vi "Verify Person as JSON.vi"(8 "error in":errorcluster) -> (0 "error out":errorcluster)   [LabVIEW 2020]
uses:
  Common/Person/Person.lvclass
  Common/Person/Person.lvclass/Person.ctl
  <vilib>/addons/_JKI Toolkits/Caraya/classes/Test/Test.lvclass
  <vilib>/SAS/Approval Tests/Extensions/Caraya.Extension/lib_Caraya.Extension.lvlib
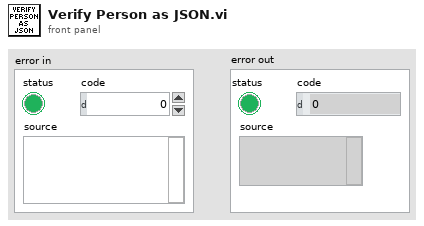
[diagram p1: front panel]
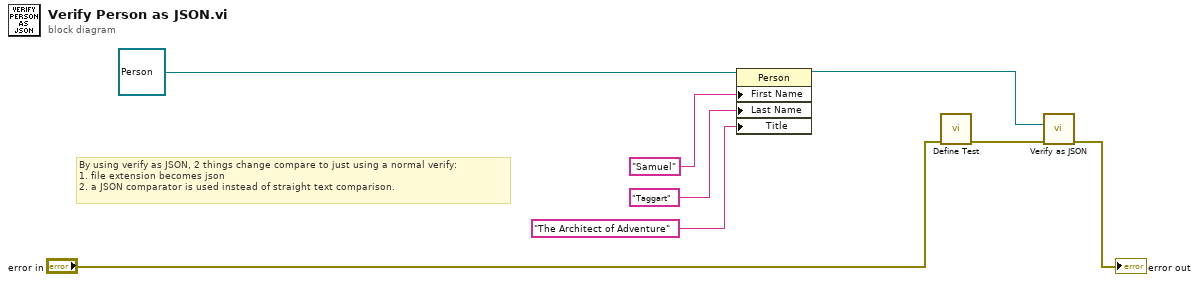
[diagram p0: block diagram]
diagram:
  # "By using verify as JSON, 2 things change compare to just using a normal verify:\n1. file extension becomes json\n2. a JSON comparator is used instead of straight text comparison."
  n1 = property class="Person"(reference=refnum<class "Person.lvclass"> refnum ("Person.lvclass"), "First Name"="Samuel", "Last Name"="Taggart", "Title"="The Architect of Adventure") -> (reference out=w1:refnum<class "Person.lvclass">)  [unwired: 1 in, 1 out]
  n2 = call <vilib>:"Define Test.vi"("error in (no error)"="error in") -> ("error out"=w8:errorcluster)  [unwired: 9 in, 1 out]
  n3 = call <vilib>:"Verify as JSON.vi"("error in"=w8, "Anything"=w1) -> ("error out"=→"error out":errorcluster)  [unwired: 8 in, 1 out]
